vi "ZE_Recorder_ReadOrPopUp.vi"(8 "error in":errorcluster, 10 "Use existing":bool, 11 "channel name":string) -> (0 "error out":errorcluster, 3 "channel config":T1)   [LabVIEW 2025, in "ZE_Recorder.lvlib"]
uses:
  ZE_Recorder.lvlib
  ZE_Recorder_TempParam.ctl
  ZE_Recorder_TempType.ctl
  ZE_Recorder_TempChannelAction.ctl
panel:
  # "Connector Pane"
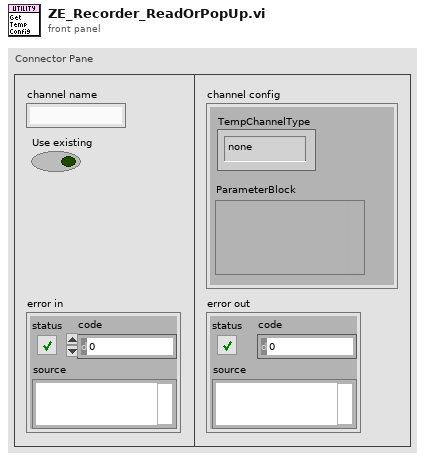
[diagram p1: front panel]
types:
  T1 = typedef "ZE_Recorder.lvlib/ZE_Recorder_TempParam.ctl" = cluster{"ParameterBlock":variant, "TempChannelType":T2}
  T2 = typedef "ZE_Recorder.lvlib/ZE_Recorder_TempType.ctl" = enum16{"none", "Thermocouple", "RTD", "Thermistor VE", "Thermistor CE"}
  T3 = typedef "ZE_Recorder.lvlib/ZE_Recorder_TempChannelAction.ctl" = enum16{"Get Channel Configs", "Read Config", "Add Config", "Clear"}
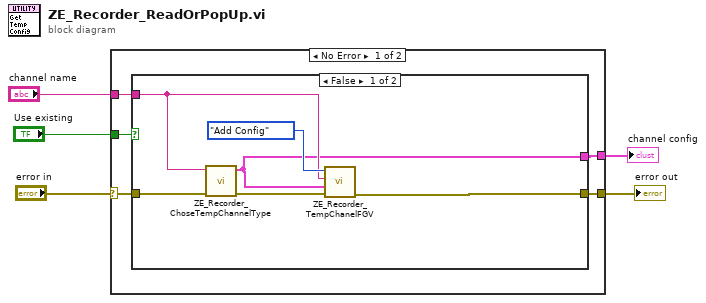
[diagram p0: block diagram]
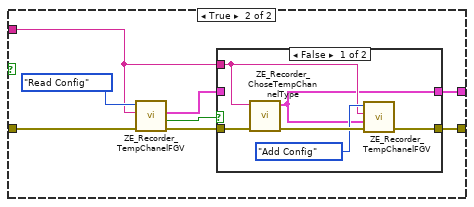
[diagram p2: hidden frame]
diagram:
  n1 = case shown="No Error" "error in" {
    selector: "error in" -> [w6 w33]
    tunnel: "Use existing" -> [w10 _]
    tunnel: "channel name" -> [w9 _]
    tunnel: [w8 _] -> w3
    tunnel: [w7 w33] -> w2
    frame No Error {
      n2 = case shown="False" w10 {
        tunnel: w6 -> [w16 w20]
        tunnel: [w11 w22] -> w8
        tunnel: w9 -> [w13 w19]
        tunnel: [w12 w17] -> w7
        frame False {
          n3 = call "ZE_Recorder_ChoseTempChannelType.vi"("error in"=w16, "channel name"=w13) -> ("error out"=w14:errorcluster, "Cluster"=w11:T1)  [unwired: 8 in]
          n4 = call "ZE_Recorder_TempChanelFGV.vi"("error in"=w14, "Config In"=w11, "channel name in"=w13, "Action"=ZE_Recorder_TempChannelAction."Add Config") -> ("error out"=w12:errorcluster)  [unwired: 4 in, 3 out]
        }
        frame True {
          n5 = call "ZE_Recorder_TempChanelFGV.vi"("error in"=w20, "channel name in"=w19, "Action"=ZE_Recorder_TempChannelAction."Read Config") -> ("error out"=w18:errorcluster, "found?"=w24:bool, "channel config"=w23:T1)  [unwired: 5 in, 1 out]
          n6 = case shown="False" w24 {
            tunnel: w23 -> [_ w32]
            tunnel: [w25 w32] -> w22
            tunnel: w19 -> [w26 _]
            tunnel: w18 -> [w30 w31]
            tunnel: [w28 w31] -> w17
            frame False {
              n7 = call "ZE_Recorder_ChoseTempChannelType.vi"("error in"=w30, "channel name"=w26) -> ("error out"=w29:errorcluster, "Cluster"=w25:T1)  [unwired: 8 in]
              n8 = call "ZE_Recorder_TempChanelFGV.vi"("error in"=w29, "Config In"=w25, "channel name in"=w26, "Action"=ZE_Recorder_TempChannelAction."Add Config") -> ("error out"=w28:errorcluster)  [unwired: 4 in, 3 out]
            }
            frame True {
            }
          }
        }
      }
    }
    frame Error {
    }
  }
  "error out" <- w2
  "channel config" <- w3
